vi "Configure Offset And Limits List (Spectrum Emissions Mask - Frequency And Bandwidth).vi"(0 "VISA resource name":refnum<visa-resource-name>, 1 "Enable Auto Resolution Bandwidth List":bool[](array[boolean])=[TRUE, TRUE], 2 "Manual Resolution Bandwidth List":dbl[](array[numeric])=[30000.0, 30000.0] format="%#.6g", 3 "Measurement Bandwidth List":dbl[](array[numeric])=[1.0, 1.0] format="%#.6g", 5 "Start Frequency State":bool[](array[boolean])=[TRUE, TRUE], 7 "Manual Start Frequency List":dbl[](array[numeric])=[2500000.0, 2500000.0] format="%#.6g", 9 "Stop Frequency List":dbl[](array[numeric])=[2715000.0, 2715000.0] format="%#.6g", 11 "error in (no error)":errorcluster, 12 "Enable Auto Sweep Time List":bool[](array[boolean])=[TRUE, TRUE], 13 "Sweep Time List":dbl[](array[numeric])=[0.008, 0.008] format="%#.6g") -> (4 "VISA resource name out":refnum<visa-resource-name>, 15 "error out":errorcluster)   [LabVIEW 2014, in "Agilent ESA PSA Series.lvlib"]
doc: "Sets the frequency, resolution bandwidth, sweep state and time for a specific offset for spectrum analyzer spectrum emission mask measurements."
uses:
  Agilent ESA PSA Series.lvlib
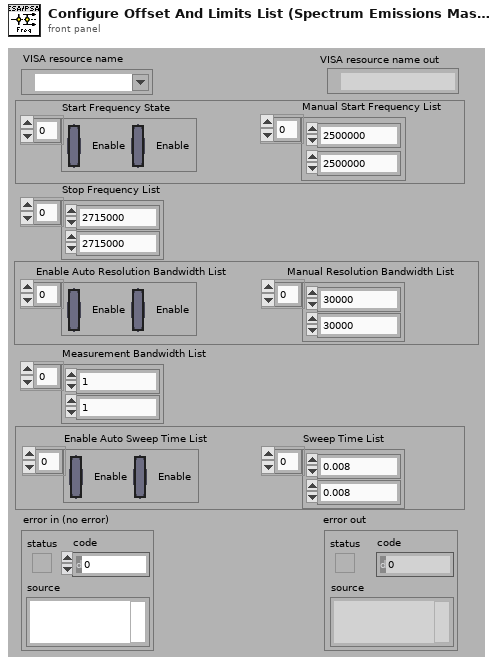
[diagram p1: front panel]
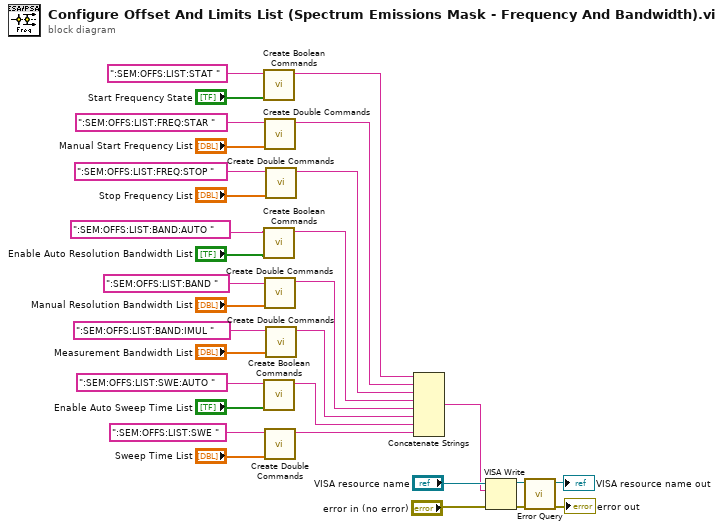
[diagram p0: block diagram]
diagram:
  n1 = call "Create Boolean Commands.vi"("States"="Start Frequency State", "Command"=":SEM:OFFS:LIST:STAT ") -> ("Result String"=w9:string)  [unwired: 9 in]
  n2 = call "Create Boolean Commands.vi"("States"="Enable Auto Resolution Bandwidth List", "Command"=":SEM:OFFS:LIST:BAND:AUTO ") -> ("Result String"=w6:string)  [unwired: 9 in]
  n3 = call "Create Boolean Commands.vi"("States"="Enable Auto Sweep Time List", "Command"=":SEM:OFFS:LIST:SWE:AUTO ") -> ("Result String"=w3:string)  [unwired: 9 in]
  n4 = call "Create Double Commands.vi"("Double Values"="Manual Start Frequency List", "Commands"=":SEM:OFFS:LIST:FREQ:STAR ") -> ("Result"=w8:string)  [unwired: 9 in]
  n5 = call "Create Double Commands.vi"("Double Values"="Manual Resolution Bandwidth List", "Commands"=":SEM:OFFS:LIST:BAND ") -> ("Result"=w5:string)  [unwired: 9 in]
  n6 = call "Create Double Commands.vi"("Double Values"="Sweep Time List", "Commands"=":SEM:OFFS:LIST:SWE ") -> ("Result"=w2:string)  [unwired: 9 in]
  n7 = call "Create Double Commands.vi"("Double Values"="Stop Frequency List", "Commands"=":SEM:OFFS:LIST:FREQ:STOP ") -> ("Result"=w7:string)  [unwired: 9 in]
  n8 = call "Create Double Commands.vi"("Double Values"="Measurement Bandwidth List", "Commands"=":SEM:OFFS:LIST:BAND:IMUL ") -> ("Result"=w4:string)  [unwired: 9 in]
  n9 = Concatenate Strings(w9, w8, w7, w6, w5, w4, w3, w2) -> (w1:string)
  n10 = VISA Write(VISA resource name="VISA resource name", write buffer=w1, error in (no error)="error in (no error)") -> (VISA resource name out=w31:refnum<visa-resource-name>, error out=w30:errorcluster)  [unwired: 1 out]
  n11 = call "Error Query.vi"("error in (no error)"=w30, "VISA resource name"=w31) -> ("error out"=→"error out":errorcluster, "VISA resource name out"=→"VISA resource name out":refnum<visa-resource-name>)  [unwired: 6 in, 2 out]
